vi "write control value.vi"(6 "call chain index (1)":i32=1, 7 "vi ref (caller)":refnum<vi>, 8 "error in (no error)":errorcluster, 10 "value":variant, 11 "label":string) -> (0 "error out":errorcluster)   [LabVIEW 2024, in "controls manager.lvlib"]
uses:
  controls manager.lvlib
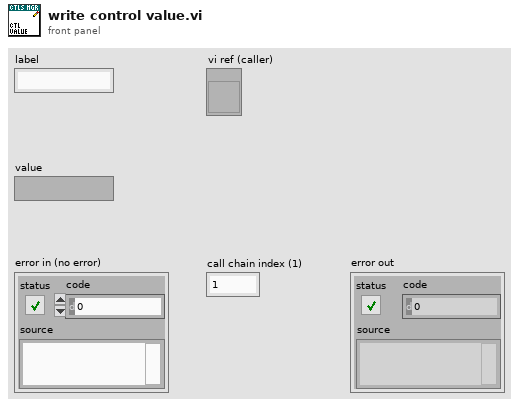
[diagram p1: front panel]
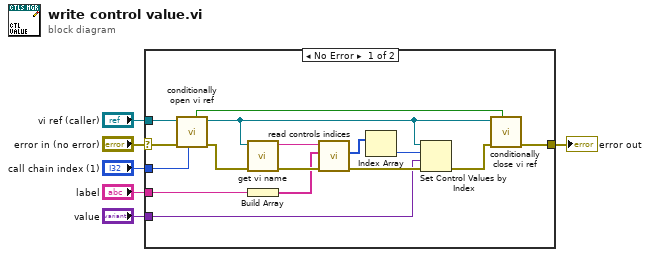
[diagram p0: block diagram]
diagram:
  n1 = case shown="No Error" "error in (no error)" {
    selector: "error in (no error)" -> [w21 w23]
    tunnel: [w18 w23] -> w6
    tunnel: "vi ref (caller)" -> [w15 _]
    tunnel: "call chain index (1)" -> [w14 _]
    tunnel: "label" -> [w13 _]
    tunnel: "value" -> [w7 _]
    frame No Error {
      n2 = call "conditionally open vi ref.vi"("call chain index (1)"=w14, "error in (no error)"=w21, "vi ref in"=w15) -> ("error out"=w20:errorcluster, "vi ref out"=w11:refnum<vi>, "new ref?"=w17:bool)  [unwired: 6 in]
      n3 = call "get vi name.vi"("error in (no error)"=w20, "vi ref"=w11) -> ("error out"=w22:errorcluster, "vi name"=w16:string)  [unwired: 8 in]
      n4 = Build Array(w13) -> (w10:string[])
      n5 = call "read controls indices.vi"("error in (no error)"=w22, "labels"=w10, "id"=w16) -> ("error out"=w19:errorcluster, "indices"=w9:i32[])  [unwired: 7 in]
      n6 = Index Array(array=w9) -> (element=w8:i32)  [unwired: 1 in]
      n7 = Set Control Values by Index(0:w11, 1:w8, 2:w7, 3:w19) -> (11:w12:errorcluster)
      n8 = call "conditionally close vi ref.vi"("new ref?"=w17, "error in (no error)"=w12, "vi ref"=w11) -> ("error out"=w18:errorcluster)  [unwired: 8 in]
    }
    frame Error {
    }
  }
  "error out" <- w6
